vi "Build Moves Map.vi"(11 "Array in":T4[](array[typedef])) -> (2 "Moves":cluster{"Action":T1, "Direction":T2}[][][](array[cluster]))   [LabVIEW 2015, in "Base Builder.lvclass"]
uses:
  Base Builder.lvclass
  Move Map Element.ctl
  Type Defs/Action Enum.ctl
  Type Defs/Direction Enum.ctl
  SubVIs/Read-Only Globals.vi
  Square/Square.lvclass
  Type Defs/SB Type Defs.lvlib
panel:
  out "x-y":dbl
  out "Moves Map":T3(array[cluster])
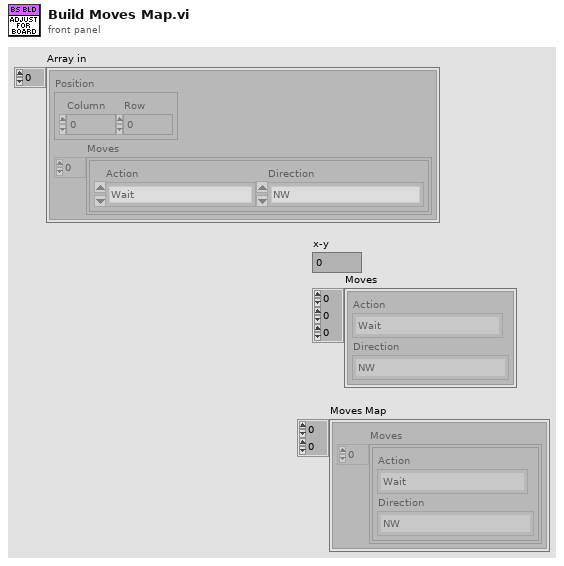
[diagram p1: front panel]
types:
  T1 = typedef "SB Type Defs.lvlib/Action Enum.ctl" = enum16{"Wait", "Move", "Attack", "Replicate"}
  T2 = typedef "SB Type Defs.lvlib/Direction Enum.ctl" = enum16{"NW", "N", "NE", "E", "SE", "S", "SW", "W"}
  T3 = cluster{"Moves":cluster{"Action":T1, "Direction":T2}[]}[][]
  T4 = typedef "Base Builder.lvclass/Move Map Element.ctl" = cluster{"Position":cluster{"Column":i32, "Row":i32}, "Moves":cluster{"Action":T1, "Direction":T2}[]}
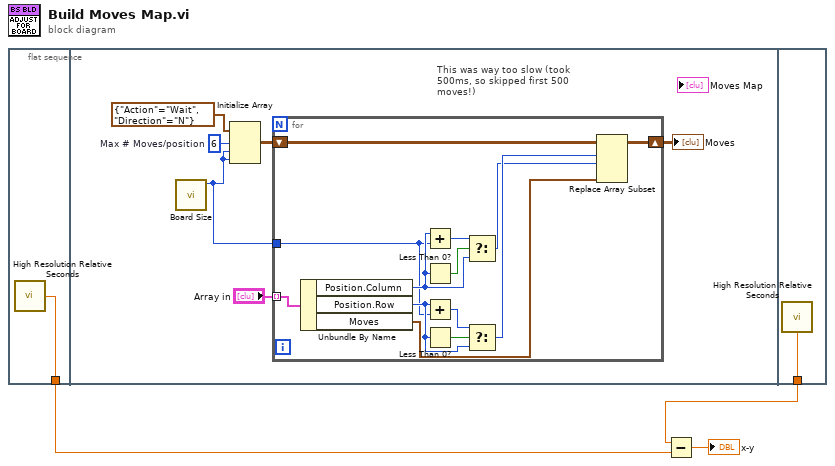
[diagram p0: block diagram]
diagram:
  n1 = flat-sequence {
    tunnel: [w4] -> w2
    tunnel: [w24] -> w3
    frame #0 {
      n2 = call <vilib>:"High Resolution Relative Seconds.vi"() -> ("relative seconds"=w4:dbl)
    }
    frame #1 {
      w6 = 6  # Max # Moves/position
      # "This was way too slow (took 500ms, so skipped first 500 moves!)"
      n3 = call "Board Size.vi"() -> ("Board Size"=w7:i32)  [unwired: 11 in]
      n4 = Initialize Array(cluster{"Action":T1, "Direction":T2} {"Action"=enum."Wait", "Direction"=enum."N"}, w6, w7, w7) -> (w5:cluster{"Action":T1, "Direction":T2}[][][])
      n5 = for {
        tunnel: "Array in" -> [w20] mode=indexing
        shift-right: [w15] -> w9
        shift-left: w5 -> [w16]
        tunnel: w7 -> [w12]
        n6 = Unbundle By Name(w20) -> ("Position.Column"=w17:i32, "Position.Row"=w21:i32, "Moves"=w11:cluster{"Action":T1, "Direction":T2}[])
        n7 = Add(x=w17, y=w12) -> (x+y=w19:i32)
        n8 = Less Than 0?(x=w17) -> (x < 0?=w18:bool)
        n9 = Add(x=w21, y=w12) -> (x+y=w22:i32)
        n10 = Less Than 0?(x=w21) -> (x < 0?=w23:bool)
        n11 = Select(t=w19, s=w18, f=w17) -> (s? t:f=w13:i32)
        n12 = Select(t=w22, s=w23, f=w21) -> (s? t:f=w14:i32)
        n13 = Replace Array Subset(array=w16, new element=w11, index (dim 0)=w14, index (dim 1)=w13) -> (w15:cluster{"Action":T1, "Direction":T2}[][][])  [unwired: 1 in]
      }
      "Moves" <- w9
    }
    frame #2 {
      n14 = call <vilib>:"High Resolution Relative Seconds.vi"() -> ("relative seconds"=w24:dbl)
    }
  }
  n15 = Subtract(x=w3, y=w2) -> (x-y=→"x-y":dbl)
